vi "FXP_Matrix-Vector_mult_loop_32bit.vi"(9 "Ns_1":u8=9, 11 "inputValid":bool) -> (2 "finished":bool)   [LabVIEW 2017]
doc: "Multiplies <B>Matrix A</B> by an input <B>Vector b</B>. This operation is useful for FPGA control applications, such as state-feedback control. You can use more than one multiplier to reduce the latency of this operation. To define <B>Matrix A</B>, double-click this Express VI and use the <B>Matrix Data Initialization</B> page to specify a VI, TXT, or CSV file that contains the matrix data. If you do not define <B>Matrix A</B>, this Express VI uses a matrix of zeroes instead.\n--------------------\n\nThis Express VI is configured as follows:\n\n<b>Fixed-Point Configuration</b>\nMatrix A Type: <+/-,32,16>\nVector b Type: <+/-,32,16>\nVector c Type: <+/-,64,36>\nOverflow mode: Truncate [Not Needed]\nRounding mode: Saturate [Not Needed]\n\n<b>Matrix A Configuration</b>\nMatrix Dimensions: 9 * 9\n\n<b>Multiplier Configuration</b>\nNumber of multipliers: 9\nNumber of multiplier pipeline stages: 0\n\n<b>Implementation</b>\nMatrix Vector Multiplication: 11 cycles"
uses:
  <vilib>/Platform/TimedLoop/XDataNode/timing_clust.ctl
  <vilib>/Platform/TimedLoop/XDataNode/nitl_modes.ctl
  <vilib>/Platform/TimedLoop/XDataNode/wakeup.ctl
  typeDefs/A_as_vec_bram.ctl
  typeDefs/x_vec_bram.ctl
  <vilib>/rvi/IPIntegrationNode/IPINode_Typedef/niFpgaIPINodeSupportedFamilies.ctl
  <vilib>/rvi/Emulation/niFpgaSctlEmulationGetInTimedLoop.vi
  <vilib>/rvi/Emulation/niFpgaEmulationReportErrorSimple.vi
  <vilib>/rvi/Emulation/niFpgaGetClockAttributes.vi
  <vilib>/rvi/Emulation/niFpgaCriticalErrorInLSC.vi
  <vilib>/rvi/IPIntegrationNode/IPINode_Utilities/niFpgaIPINodeSimCore.vi
  <vilib>/rvi/DataTransferAndStorage/Container/Common/niFpgaContainerExecOnDevCompGetState.vi
  <vilib>/rvi/Emulation/niFpgaEmulationIsFPGAContextNoSignature.vi
  <vilib>/rvi/DataTransferAndStorage/Container/Common/niFpgaContainerGetUniqueNameForEmu.vi
  <vilib>/rvi/Emulation/niFpgaProcessEmulError.vi
  <vilib>/rvi/errors/nirviReportUnexpectedCaseInternalError (U32).vi
  <vilib>/rvi/Memory/Memory_Emulation/niFpgaMemoryEmulationCacheClearOnFirstRun.vi
  <vilib>/rvi/Memory/Memory_Emulation/nirvimemoryEmulationManagerCache_MakeExclusive.vi
  <vilib>/rvi/Memory/Memory_Emulation/niFpgaMemoryEmulationValidateCache.vi
  <vilib>/rvi/Memory/Memory_Emulation/nirvimemoryEmulationManagerCache_InsertValue.vi
  <vilib>/Utility/error.llb/Clear Errors.vi
  <vilib>/rvi/Memory/Memory_Emulation/nirvimemoryEmulationManagerCache_ReleaseExclusive.vi
  <vilib>/rvi/Memory/Memory_Emulation/nirvimemoryEmulationManagerCache_GetValue.vi
  <vilib>/rvi/Memory/Memory_Emulation/nirvimemoryEmulationManagerCache_SetValue.vi
  <vilib>/rvi/Emulation/niFpgaSctlEmulationResourceMgr.vi
  <vilib>/Platform/TimedLoop/XDataNode/XDataNode.xnode
  <vilib>/rvi/XilinxIP/XIPIN_XNode/niFpgaXIPIN.xnode
  MAC01 1/MAC01_1_75F243352369479695E2AED5F4206BF1.dll
  <vilib>/rvi/IPIntegrationNode/IPINode_Xnode/niFpgaIPINode.xnode
  <vilib>/rvi/DataTransferAndStorage/Container/XNode/niFpgaContainer.xnode
  <vilib>/rvi/Memory/Memory_Emulation/niFpgaMemoryEmulationRefIn.vi
  <vilib>/Platform/TimedLoop/XDataNode/XDNodeRunTimeDep.lvlib
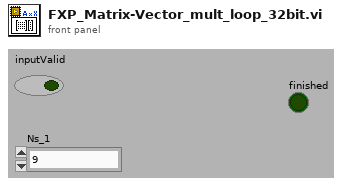
[diagram p1: front panel]
types:
  T1 = typedef "x_vec_bram.ctl" = refnum<k21>
  T2 = typedef "A_as_vec_bram.ctl" = refnum<k21>
  T3 = typedef "XDNodeRunTimeDep.lvlib/timing_clust.ctl" = cluster{"Expected End [f-1]":u64, "Actual End [f-1]":u64, "Finished Late? [f-1]":bool, "Expected End [i-1]":u64, "Actual End [i-1]":u64, "Finished Late? [i-1]":bool, "Expected Start [i]":u64, "Actual Start [i]":u64, "Expected Start [f]":u64, "Actual Start [f]":u64, "Source Name":string, "Structure Name":string, "Period":i64, "Deadline":i64, "Offset":i64, "Start":i64, "Priority":i32, "Timeout":i32, "Mode":T4, "Wakeup Reason":T5, "Error":errorcluster, "Source Type":string, "Secondary Source Type":string, "Global End Time":u64, "Global Start Time":u64, "Frame Duration":u64, "Iteration Duration":u64, "Assigned CPU":i32, "I/O Scan Engine Mode":u32}
  T4 = typedef "XDNodeRunTimeDep.lvlib/nitl_modes.ctl" = enum32{"No Change", "Process missed periods, maintain original phase", "Discard missed periods, maintain original phase", "Process missed periods, ignore original phase", "Discard missed periods, ignore original phase"}
  T5 = typedef "XDNodeRunTimeDep.lvlib/wakeup.ctl" = enum32{"Normal", "Aborted", "Asynchronous wakeup", "Timing source error", "Timed loop error", "Timeout"}
  T6 = typedef "niFpgaIPINodeSupportedFamilies.ctl" = cluster{"unlimited?":bool, "supported targets":string[]}
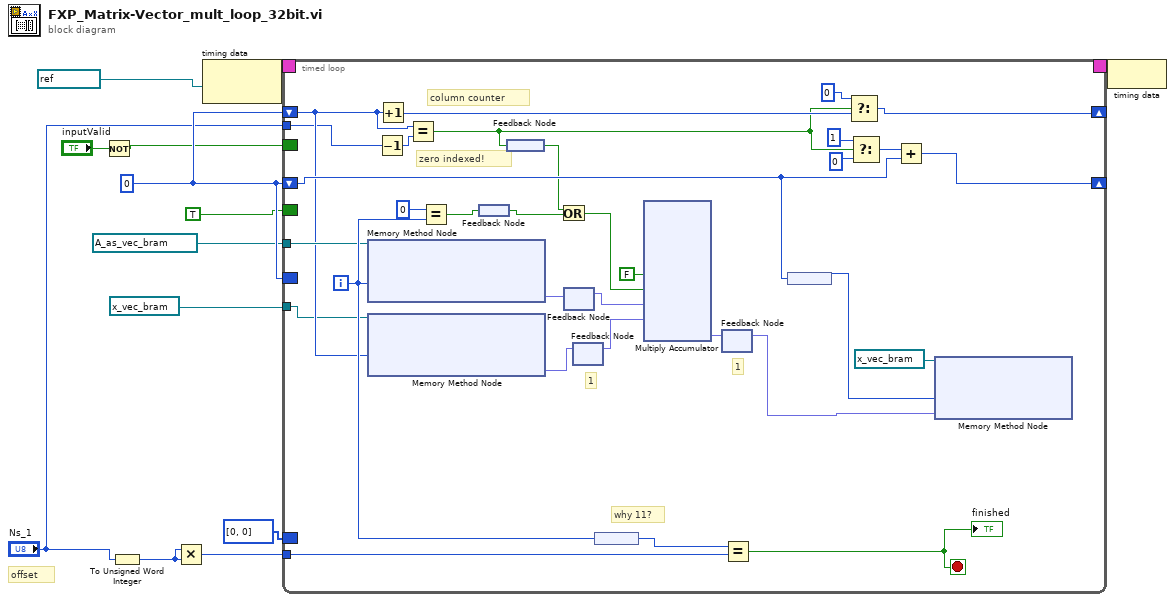
[diagram p0: block diagram]
diagram:
  w11 = u8 0
  # "offset"
  n1 = Not(x="inputValid") -> (.not. x?=w8:bool)
  n2 = To Unsigned Word Integer(number="Ns_1") -> (unsigned 16bit integer=w10:u16)
  n3 = Multiply(x=w10, y=w10) -> (x*y=w5:u16)
  n4 = node-c288(refnum<k21> "80MHz" ("Source Name")) -> (w13:T3)
  n5 = timed-loop {
    timing: w13 -> [_]
    timing-out: [_] -> w12
    shift-right: [w40] -> _
    shift-left: w11 -> [w37]
    shift-right: [w44] -> _
    shift-left: w11 -> [w26]
    border: w8 -> [_]
    border: w11 -> [_]
    tunnel: T2 "AasCol _FXP" ("Memory In") -> [w28]
    tunnel: w5 -> [w27]
    tunnel: T1 "xk_0_1" ("Memory") -> [w25]
    border: TRUE -> [_]
    border: i32[] [0, 0] -> [_]
    tunnel: "Ns_1" -> [w22]
    i -> [w30]
    stop <- w45 stop-if-true
    # "why 11?"
    # "1"
    # "1"
    # "zero indexed!"
    # "column counter"
    n6 = xnode ("Memory Method Node")("Address"=w30, "Memory In"=w28) -> ("Data"=w21:fxp<+/-,32,7>)  [unwired: 1 out]
    n7 = xnode ("Memory Method Node")("Address"=w26, "Memory In"=w25) -> ("Data"=w18:fxp<+/-,32,6>)  [unwired: 1 out]
    n8 = Decrement(x=w22) -> (x-1=w35:u8)
    n9 = Increment(x=w26) -> (x+1=w39:u8)
    n10 = Equal?(x=w26, y=w35) -> (x = y?=w36:bool)
    n11 = Equal?(x=0, y=w30) -> (x = y?=w23:bool)
    n12 = feedback #1() -> (w24:bool)
    n13 = feedback-in #1(w23) -> ()
    n14 = feedback #2() -> (w34:bool)
    n15 = feedback-in #2(w36) -> ()
    n16 = Or(x=w34, y=w24) -> (x .or. y?=w33:bool)
    n17 = feedback-in #3(w21) -> ()
    n18 = feedback #3() -> (w20:fxp<+/-,32,7>)  [unwired: 1 in]
    n19 = feedback #4() -> (w19:fxp<+/-,32,6>)  [unwired: 1 in]
    n20 = feedback-in #4(w18) -> ()
    n21 = feedback #5() -> (w31:i32)
    n22 = feedback-in #5(w30) -> ()
    n23 = xnode ("Multiply Accumulator")("sclr"=FALSE, "bypass"=w33, "a"=w20, "b"=w19) -> ("s"=w17:fxp<+/-,36,13>)  [unwired: 1 in]
    n24 = feedback #6() -> (w14:fxp<+/-,36,13>)  [unwired: 1 in]
    n25 = feedback-in #6(w17) -> ()
    n26 = Equal?(x=w31, y=w27) -> (x = y?=w45:bool)
    "finished" <- w45
    n27 = feedback #7() -> (w15:u8)
    n28 = feedback-in #7(w37) -> ()
    n29 = Select(t=u8 0, s=w36, f=w39) -> (s? t:f=w44:u8)
    n30 = Select(t=u8 1, s=w36, f=u8 0) -> (s? t:f=w41:u8)
    n31 = Add(x=w41, y=w37) -> (x+y=w40:u8)
    n32 = xnode ("Memory Method Node")("Address"=w15, "Data"=w14, "Memory In"=T1 "xk_1_0" ("Memory")) -> ()  [unwired: 1 out]
  }
  n33 = node-c288(w12) -> ()
